vi "Write System Friction.vi"(6 "error in":errorcluster, 8 "MaxRead":i32, 9 "Channel in":u16) -> (0 "error out":errorcluster, 1 "Messages":T1(array[cluster]), 2 "Pass":bool, 3 "Channel out":u16)   [LabVIEW 2023]
uses:
  be2a90bf-c340-472d-9dbd-2edbd756b5ea.vi
  25c4d7a5-05b7-46bb-9aa9-728f7a481570.vi
  Communication/PCAN2023/PCAN API.lvlib
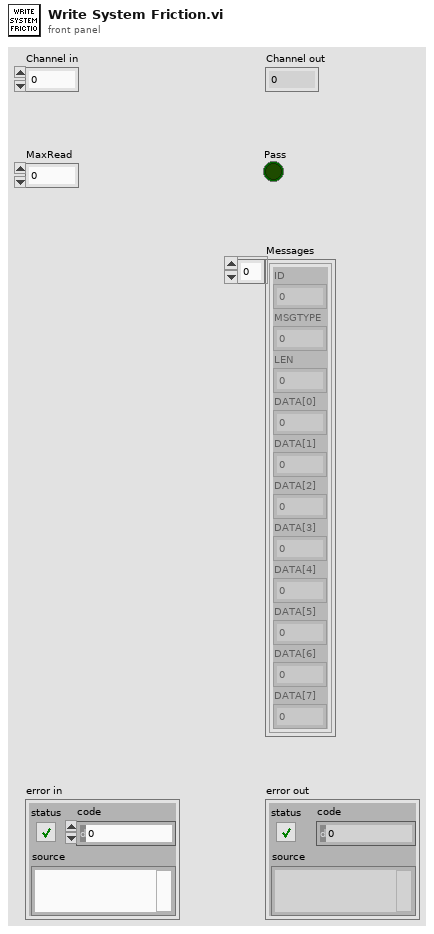
[diagram p1: front panel]
types:
  T1 = cluster{"ID":u32, "MSGTYPE":u8, "LEN":u8, "DATA[0]":u8, "DATA[1]":u8, "DATA[2]":u8, "DATA[3]":u8, "DATA[4]":u8, "DATA[5]":u8, "DATA[6]":u8, "DATA[7]":u8}[]
  T2 = cluster{"ID":u32, "MSGTYPE":u8, "LEN":u8, "DATA[0]":u8, "DATA[1]":u8, "DATA[2]":u8, "DATA[3]":u8, "DATA[4]":u8, "DATA[5]":u8, "DATA[6]":u8, "DATA[7]":u8}
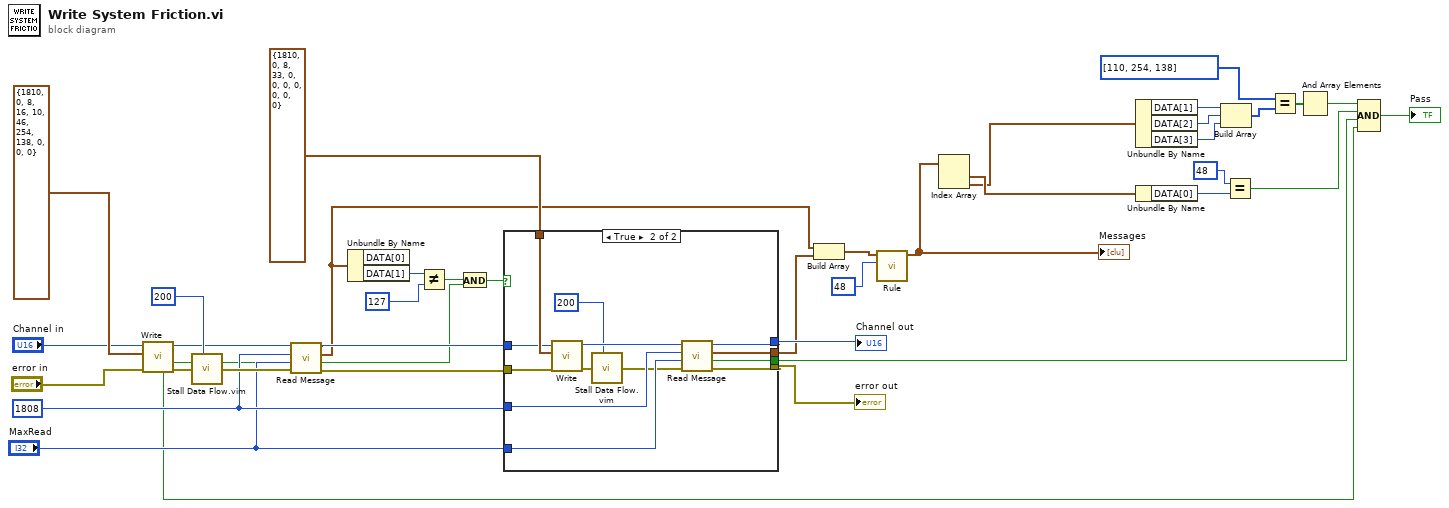
[diagram p0: block diagram]
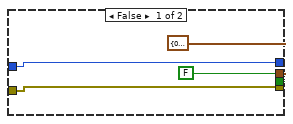
[diagram p2: hidden frame]
diagram:
  w13 = u32 1808 ("ID")
  n1 = call "Write.vi"("error in"="error in", "MessageBuffer"=T2 {"ID"=1810, "MSGTYPE"=0, "LEN"=8, "DATA[0]"=16, "DATA[1]"=10, "DATA[2]"=46, "DATA[3]"=254, "DATA[4]"=138, "DATA[5]"=0, "DATA[6]"=0, "DATA[7]"=0}, "Channel"="Channel in") -> ("error out"=w37:errorcluster, "Channel out"=w18:u16)  [unwired: 5 in, 2 out]
  n2 = call "Stall Data Flow.vim"("value in"=w37, "milliseconds to wait"=u32 200) -> ("value out"=w16:errorcluster)  [unwired: 1 out]
  n3 = call "Read Message.vi"("error in"=w16, "MaxRead"="MaxRead", "ID"=w13, "Channel in"=w18) -> ("error out"=w15:errorcluster, "Passed"=w8:bool, "Last Message"=w14:T2, "Channel out"=w17:u16)  [unwired: 3 in, 1 out]
  n4 = Unbundle By Name(w14) -> ("DATA[1]"=w19:u8)  [unwired: 1 out]
  n5 = Not Equal?(x=w19, y=u8 127) -> (x != y?=w5:bool)
  n6 = And(x=w5, y=w8) -> (x .and. y?=w9:bool)
  n7 = case shown="True" w9 {
    tunnel: T2 {"ID"=1810, "MSGTYPE"=0, "LEN"=8, "DATA[0]"=33, "DATA[1]"=0, "DATA[2]"=0, "DATA[3]"=0, "DATA[4]"=0, "DATA[5]"=0, "DATA[6]"=0, "DATA[7]"=0} ("MessageBuffer") -> [_ w55]
    tunnel: w17 -> [w42 w54]
    tunnel: w15 -> [w41 w53]
    tunnel: [w41 w49] -> w25
    tunnel: w13 -> [_ w47]
    tunnel: [w42 w51] -> w22
    tunnel: [T2 {"ID"=0, "MSGTYPE"=0, "LEN"=0, "DATA[0]"=0, "DATA[1]"=0, "DATA[2]"=0, "DATA[3]"=0, "DATA[4]"=0, "DATA[5]"=0, "DATA[6]"=0, "DATA[7]"=0} ("MessageBuffer out") w50] -> w21
    tunnel: "MaxRead" -> [_ w46]
    tunnel: [FALSE ("Passed") w45] -> w10
    frame False {
    }
    frame True {
      n8 = call "Write.vi"("error in"=w53, "MessageBuffer"=w55, "Channel"=w54) -> ("error out"=w48:errorcluster, "Channel out"=w52:u16)  [unwired: 5 in, 2 out]
      n9 = call "Stall Data Flow.vim"("value in"=w48, "milliseconds to wait"=u32 200) -> ("value out"=w44:errorcluster)  [unwired: 1 out]
      n10 = call "Read Message.vi"("error in"=w44, "MaxRead"=w46, "ID"=w47, "Channel in"=w52) -> ("error out"=w49:errorcluster, "Passed"=w45:bool, "Last Message"=w50:T2, "Channel out"=w51:u16)  [unwired: 3 in, 1 out]
    }
  }
  "error out" <- w25
  "Channel out" <- w22
  n11 = Build Array(w14, w21) -> (w4:T1)
  n12 = call "Rule.vi"("Case"=u8 48 ("x"), "Array in"=w4) -> ("Array out"=w3:T1)  [unwired: 9 in]
  "Messages" <- w3
  n13 = Index Array(array=w3) -> (element #1=w7:T2, element #2=w6:T2)  [unwired: 2 in]
  n14 = Unbundle By Name(w6) -> ("DATA[1]"=w31:u8, "DATA[2]"=w30:u8, "DATA[3]"=w29:u8)
  n15 = Unbundle By Name(w7) -> ("DATA[0]"=w23:u8)
  n16 = Build Array(w31, w30, w29) -> (w28:u8[])
  n17 = Equal?(x=u8 48, y=w23) -> (x = y?=w11:bool)
  n18 = Equal?(x=u8[] [110, 254, 138], y=w28) -> (x = y?=w33:bool[])
  n19 = And Array Elements(Boolean array=w33) -> (logical AND=w27:bool)
  n20 = Compound Arithmetic op=AND(w27, w11, w10, w8) -> (→"Pass":bool)
